vi "PH_USB600x_AnalogReader.check GUI Refs.vi"(0 "i ref in":refnum<vi>, 5 "error in (no error)":errorcluster) -> (14 "i ref out":refnum<vi>, 16 "Timeout":bool, 19 "error out":errorcluster)   [LabVIEW 2014, in "PH_USB600x_AnalogReader.lvlib"]
doc: "This VI waits for the GUI indicator object refereces."
uses:
  PH_USB600x_AnalogReader.lvlib
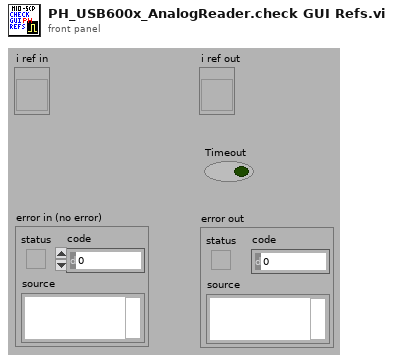
[diagram p1: front panel]
types:
  T1 = typedef "PH_USB600x_AnalogReader.lvlib/PH_USB600x_AnalogReader.i attribute.ctl" = cluster{"GUI Refs":cluster{"Delete":refnum<vi>, "Status":refnum<vi>, "Timeout":refnum<vi>, "Acquire Waveform":refnum<vi>, "Timing":refnum<vi>, "Graph":refnum<vi>, "Prdc Interval":refnum<vi>, "Formula":refnum<vi>}, "Device Settings":cluster{"AIChannel":refnum<k21>, "channelName":string, "Status":T2}, "Timing":T3, "Prdc Interval":dbl, "Lin Scaling":T4, "Data":cluster{"t0":timestamp, dbl}[]}
  T2 = typedef "PH_StatusHandler.lvlib/PH_StatusHandler.Status.ctl" = i16
  T3 = typedef "PH_USB600x_AnalogReader.lvlib/PH_USB600x_AnalogReader.Timing.ctl" = cluster{"Samples per Channel":i32, "Rate":dbl}
  T4 = typedef "PH_USB600x_AnalogReader.lvlib/PH_USB600x_AnalogReader.Lin Scaling.ctl" = cluster{"Slope [Unit/V]":dbl, "Offset [Unit]":dbl, "Y-Unit":string, "Y-Label":string}
  T5 = cluster{"Delete":refnum<vi>, "Status":refnum<vi>, "Timeout":refnum<vi>, "Acquire Waveform":refnum<vi>, "Timing":refnum<vi>, "Graph":refnum<vi>, "Prdc Interval":refnum<vi>, "Formula":refnum<vi>}
  T6 = cluster{"Delete":bool, "Status":bool, "Timeout":bool, "Acquire Waveform":bool, "Timing":bool, "Graph":bool, "Prdc Interval":bool, "Formula":bool}
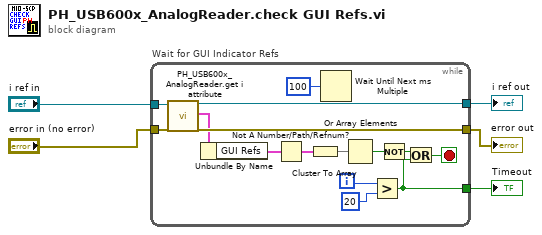
[diagram p0: block diagram]
diagram:
  n1 = while "Wait for GUI Indicator Refs" {
    tunnel: [w16] -> w2
    tunnel: [w17] -> w5
    tunnel: "error in (no error)" -> [w15]
    tunnel: "i ref in" -> [w14]
    tunnel: [w13] -> w4
    i -> [w19]
    stop <- w12 stop-if-true
    n2 = call "PH_USB600x_AnalogReader.get i attribute.vi"("i ref in"=w14, "error in (no error)"=w15) -> ("i ref out"=w13:refnum<vi>, "i attribute"=w11:T1, "error out"=w17:errorcluster)  [unwired: 15 in]
    n3 = Unbundle By Name(w11) -> ("GUI Refs"=w10:T5)
    n4 = Not A Number/Path/Refnum?(number/path/refnum=w10) -> (NaN/Path/Refnum?=w9:T6)
    n5 = Cluster To Array(cluster=w9) -> (array=w8:bool[])
    n6 = Wait Until Next ms Multiple(millisecond multiple=u32 100) -> ()  [unwired: 1 out]
    n7 = Or Array Elements(Boolean array=w8) -> (logical OR=w7:bool)
    n8 = Greater?(x=w19, y=20) -> (0:w16:bool)
    n9 = Not(x=w7) -> (.not. x?=w6:bool)
    n10 = Or(x=w6, y=w16) -> (x .or. y?=w12:bool)
  }
  "error out" <- w5
  "i ref out" <- w4
  "Timeout" <- w2
